vi "Parse Monitor Record.vi"(10 "header size bytes (32)":i32=32, 11 "Record In":u8[](array[numeric])) -> (0 "FrameHeaderInfo":T2 {"FHW0"."MacID" format="%03b"}, 1 "BECW":T7, 2 "Payload":u8[](array[numeric]) format="%.0x", 3 "Record Out":u8[](array[numeric]), 4 "IrigTime":T6, 6 "conversion time uS":u32)   [LabVIEW 2020, in "AIM664LV.lvlib"]
uses:
  AIM664LV.lvlib
  _controls/monitor_becw_type.ctl
  bsp/AFDX_Controls/IrigTime.ctl
  _controls/monitor_fhInfol_type.ctl
  _controls/monitor_entrySize_type.ctl
  _controls/monitor_fhw0_type.ctl
  _controls/monitor_fhw1_type.ctl
panel:
  in  "byte order (0:big-endian, network order)":T1(ring)=enum."native, host order"
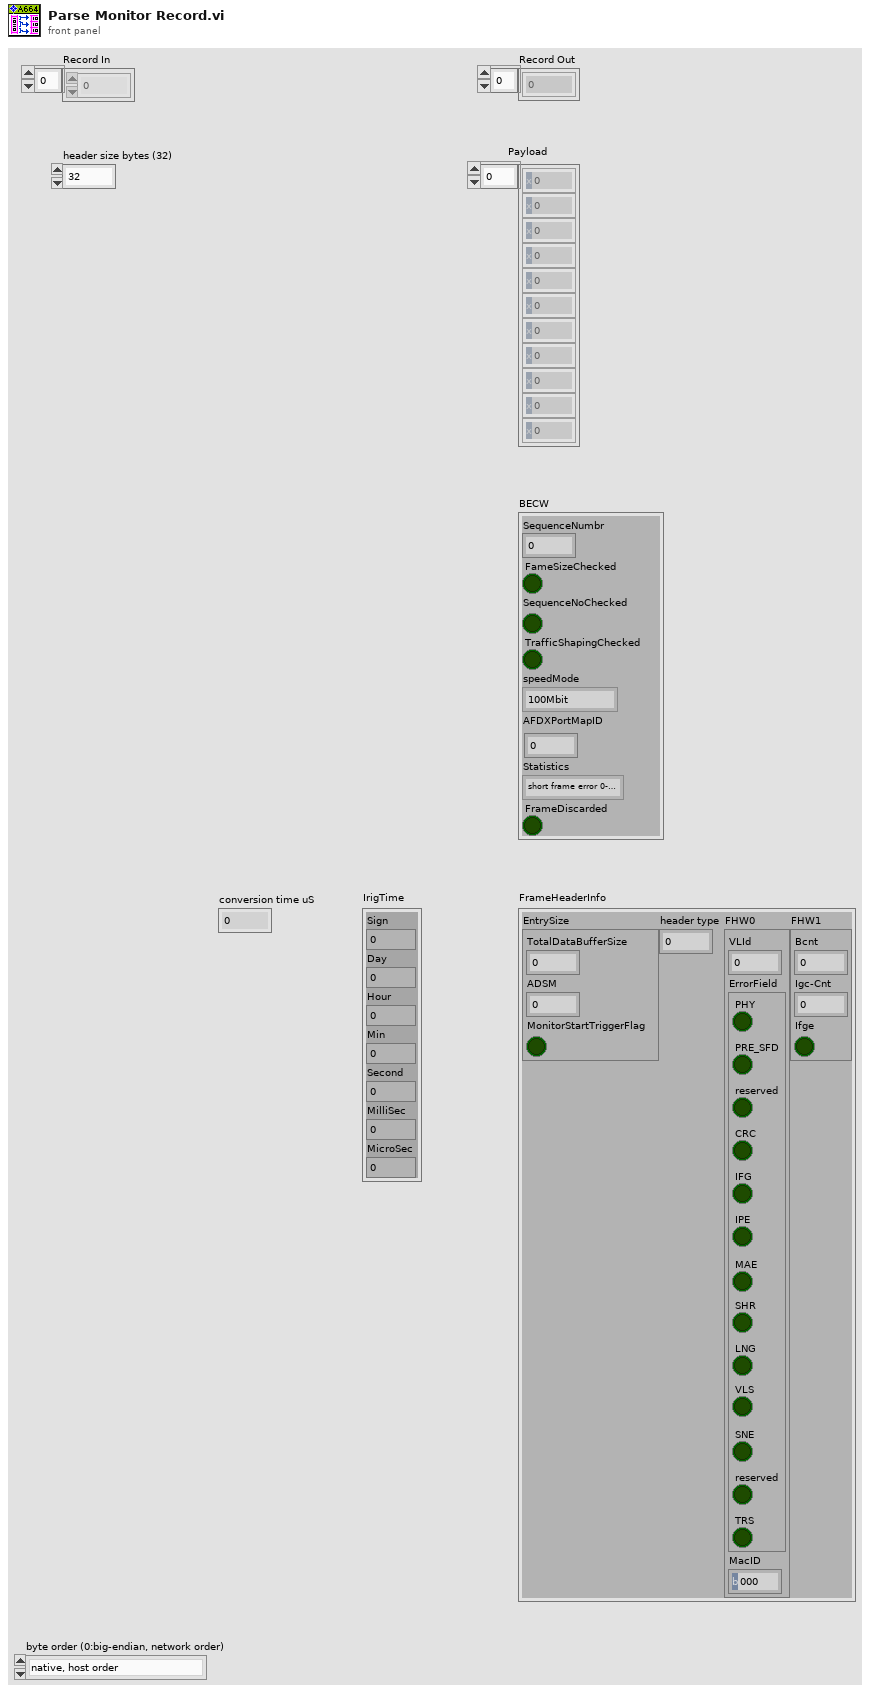
[diagram p1: front panel]
types:
  T1 = enum16{"big-endian, network order", "native, host order", "little-endian"}
  T2 = typedef "AIM664LV.lvlib/monitor_fhInfol_type.ctl" = cluster{"EntrySize":T3, "header type":u32, "FHW0":T4, "FHW1":T5}
  T3 = typedef "AIM664LV.lvlib/monitor_entrySize_type.ctl" = cluster{"TotalDataBufferSize":u16, "ADSM":u16, "MonitorStartTriggerFlag":bool}
  T4 = typedef "AIM664LV.lvlib/monitor_fhw0_type.ctl" = cluster{"VLId":u16, "ErrorField":cluster{"PHY":bool, "PRE_SFD":bool, "reserved":bool, "CRC":bool, "IFG":bool, "IPE":bool, "MAE":bool, "SHR":bool, "LNG":bool, "VLS":bool, "SNE":bool, "reserved":bool, "TRS":bool}, "MacID":u8}
  T5 = typedef "AIM664LV.lvlib/monitor_fhw1_type.ctl" = cluster{"Bcnt":u16, "Igc-Cnt":u16, "Ifge":bool}
  T6 = typedef "AIM664LV.lvlib/IrigTime.ctl" = cluster{"Sign":i32, "Day":u32, "Hour":u32, "Min":u32, "Second":u32, "MilliSec":u32, "MicroSec":u32}
  T7 = typedef "AIM664LV.lvlib/monitor_becw_type.ctl" = cluster{"SequenceNumbr":u8, "FameSizeChecked":bool, "SequenceNoChecked":bool, "TrafficShapingChecked":bool, "speedMode":enum16{"100Mbit", "10Mbit", "1Gbit"}, "AFDXPortMapID":u8, "Statistics":enum16{"short frame error 0-63Bytes", "64-127 Bytes", "128-255 Bytes", "256-511 Bytes", "512-1023 Bytes", "1024-1518 Bytes", ">1518 Bytes"}, "FrameDiscarded":bool}
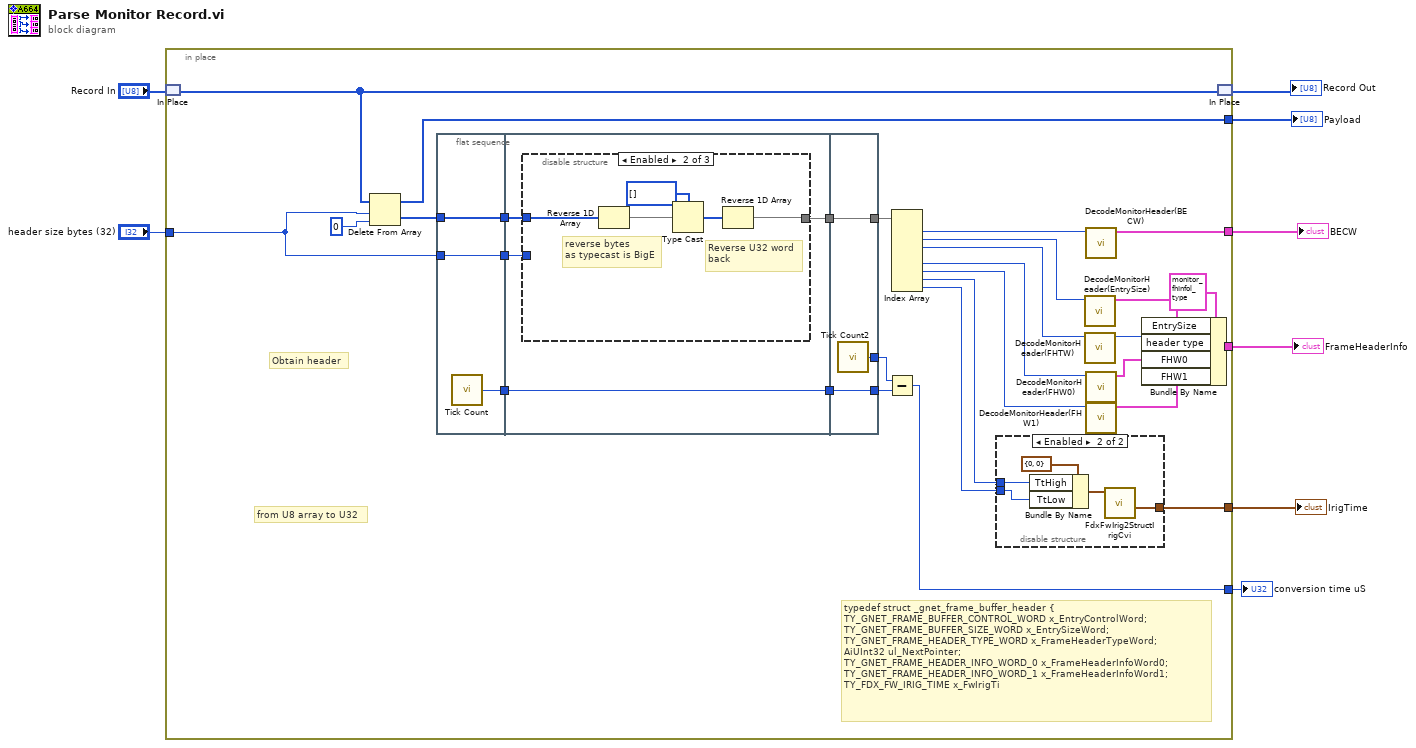
[diagram p0: block diagram]
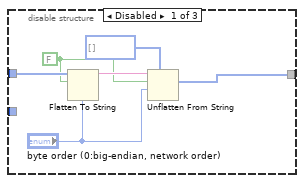
[diagram p2: hidden frame]
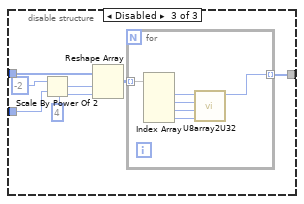
[diagram p3: hidden frame]
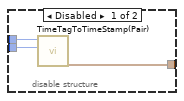
[diagram p4: hidden frame]
diagram:
  n1 = in-place {
    in-place-border: [w37] -> w8
    in-place-border: [w36] -> w7
    in-place-border: [w33] -> w6
    in-place-border: [w30] -> w5
    in-place-border: "header size bytes (32)" -> [w16]
    in-place-border: [w20] -> w1
    # "typedef struct _gnet_frame_buffer_header {\nTY_GNET_FRAME_BUFFER_CONTROL_WORD x_EntryControlWord;\nTY_GNET_FRAME_BUFFER_SIZE_WORD x_EntrySizeWord;\nTY_GNET_FRAME_HEADER_TYPE_WORD x_FrameHeaderTypeWord;\nAiUInt32 ul_NextPointer;\nTY_GNET_FRAME_HEADER_INFO_WORD_0 x_FrameHeaderInfoWord0;\nTY_GNET_FRAME_HEADER_INFO_WORD_1 x_FrameHeaderInfoWord1;\nTY_FDX_FW_IRIG_TIME x_FwIrigTi"
    # "from U8 array to U32"
    # "Obtain header"
    n2 = in-place-match #1("Record In") -> (w29:u8[])
    n3 = Delete From Array(array=w29, length=w16, index=0) -> (deleted portion=w32:u8[], array with subset deleted=w33:u8[])
    n4 = flat-sequence {
      tunnel: w32 -> [w40]
      tunnel: [w40] -> w26
      tunnel: [w39] -> w21
      tunnel: [w38] -> w17
      tunnel: w16 -> [w38]
      tunnel: w26 -> [w43]
      tunnel: [w44] -> w25
      tunnel: [w42] -> w22
      tunnel: w21 -> [w42]
      tunnel: w17 -> [w41]
      tunnel: [w71] -> w35
      tunnel: w25 -> [w71]
      tunnel: [w70] -> w24
      tunnel: [w69] -> w23
      tunnel: w22 -> [w69]
      frame #0 {
        n5 = call "Tick Count"() -> ("Tick Count(uSec)"=w39:u32)
      }
      frame #1 {
        n6 = disable-structure shown="Enabled" {
          disable-tunnel: [w47 w51 w60] -> w44
          disable-tunnel: w43 -> [w50 w55 w62]
          disable-tunnel: w41 -> [_ _ w56]
          frame Disabled {
            w46 = FALSE ("prepend array or string size? (T)")
            n7 = Flatten To String(anything=w50, prepend array or string size? (T)=w46, byte order (0:big-endian, network order)="byte order (0:big-endian, network order)") -> (data string=w48:string)  [unwired: 1 in, 2 out]
            n8 = Unflatten From String(type=u32[] [] ("index"), binary string=w48, data includes array or string size? (T)=w46, byte order (0:big-endian, network order)="byte order (0:big-endian, network order)") -> (value=w47:u32[])  [unwired: 1 in, 2 out]
          }
          frame Enabled {
            # "Reverse U32 word\nback"
            # "reverse bytes\nas typecast is BigE"
            n9 = Reverse 1D Array(array=w55) -> (reversed array=w54:u8[])
            n10 = Type Cast(type=u32[] [] ("index"), x=w54) -> (*(type *) &x=w52:u32[])
            n11 = Reverse 1D Array(array=w52) -> (reversed array=w51:u32[])
          }
          frame Disabled {
            n12 = Scale By Power Of 2(n=i16 -2, x=w56) -> (x*2^n=w57:i32)
            n13 = Reshape Array(w62, w57, i16 4 ("n")) -> (w61:u8[][])
            n14 = for {
              tunnel: w61 -> [w68] mode=indexing
              tunnel: [w63] -> w60 mode=indexing
              n15 = Index Array(array=w68) -> (element #1=w67:u8, element #2=w66:u8, element #3=w65:u8, element #4=w64:u8)  [unwired: 4 in]
              n16 = call "U8array2U32.vi"("hi 2"=w64, "lo 2"=w65, "hi"=w66, "lo"=w67) -> ("(hi.lo)"=w63:u32)  [unwired: 7 in]
            }
          }
        }
      }
      frame #2 {
        n17 = call "Tick Count2"() -> ("Tick Count(uSec)"=w70:u32)
      }
    }
    n18 = Subtract(x=w24, y=w23) -> (x-y=w20:u32)
    n19 = Index Array(array=w35) -> (element #1=w15:u32, element #2=w10:u32, element #3=w11:u32, element #5=w18:u32, element #6=w19:u32, element #7=w28:u32, element #8=w27:u32)  [unwired: 8 in, 1 out]
    n20 = disable-structure shown="Enabled" {
      disable-tunnel: [w74 w77] -> w36
      disable-tunnel: w27 -> [w73 w75]
      disable-tunnel: w28 -> [w72 w76]
      frame Disabled {
        n21 = call "TimeTagToTimeStamp(Pair).vi"("ttlw"=w73, "tthw"=w72) -> ("IrigTime"=w74:T6)  [unwired: 7 in, 2 out]
      }
      frame Enabled {
        n22 = Bundle By Name(cluster=cluster{"TtHigh":u32, "TtLow":u32} {"TtHigh"=0, "TtLow"=0} ("FwIrigTime"), "TtHigh"=w76, "TtLow"=w75) -> (w78:cluster{"TtHigh":u32, "TtLow":u32})
        n23 = call "FdxFwIrig2StructIrigCvi.vi"("FwIrigTime"=w78) -> ("IrigTime"=w77:T6)  [unwired: 9 in, 1 out]
      }
    }
    n24 = call "DecodeMonitorHeader(EntrySize).vi"("EntrySizeWord"=w10) -> ("EntrySize"=w9:T3)  [unwired: 10 in]
    n25 = call "DecodeMonitorHeader(FHTW).vi"("fhtw"=w11) -> ("header type"=w12:u32)  [unwired: 10 in]
    n26 = call "DecodeMonitorHeader(BECW).vi"("becw"=w15) -> ("BECW"=w37:T7)  [unwired: 10 in]
    n27 = call "DecodeMonitorHeader(FHW0).vi"("fhw0"=w18) -> ("FHW0"=w13:T4)  [unwired: 10 in]
    n28 = call "DecodeMonitorHeader(FHW1).vi"("fhw1"=w19) -> ("FHW1"=w14:T5)  [unwired: 10 in]
    n29 = Bundle By Name(cluster=T2 {"EntrySize"={"TotalDataBufferSize"=0, "ADSM"=0, "MonitorStartTriggerFlag"=FALSE}, "header type"=0, "FHW0"={"VLId"=0, "ErrorField"={"PHY"=FALSE, "PRE_SFD"=FALSE, "reserved"=FALSE, "CRC"=FALSE, "IFG"=FALSE, "IPE"=FALSE, "MAE"=FALSE, "SHR"=FALSE, "LNG"=FALSE, "VLS"=FALSE, "SNE"=FALSE, "reserved"=FALSE, "TRS"=FALSE}, "MacID"=0}, "FHW1"={"Bcnt"=0, "Igc-Cnt"=0, "Ifge"=FALSE}} ("FrameHeaderInfo"), "EntrySize"=w9, "header type"=w12, "FHW0"=w13, "FHW1"=w14) -> (w30:T2)
    n30 = in-place-match #1(w29) -> (→"Record Out":u8[])
  }
  "IrigTime" <- w7
  "BECW" <- w8
  "FrameHeaderInfo" <- w5
  "Payload" <- w6
  "conversion time uS" <- w1
